vi "check upper bound.vi"(8 "error in (no error)":errorcluster, 9 "ptr upper bound (inclusive)":u64, 10 "size":u64, 11 "ptr in":u64) -> (0 "error out":errorcluster)   [LabVIEW 2018, in "linuxSharedMemory.lvlib"]
uses:
  linuxSharedMemory.lvlib
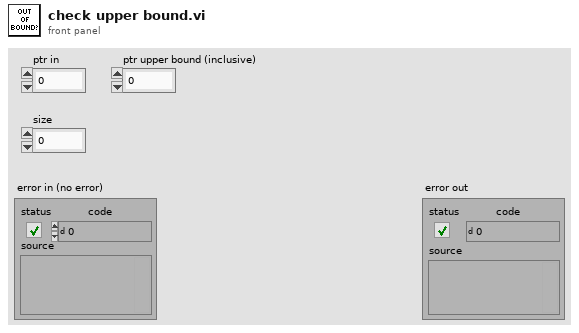
[diagram p1: front panel]
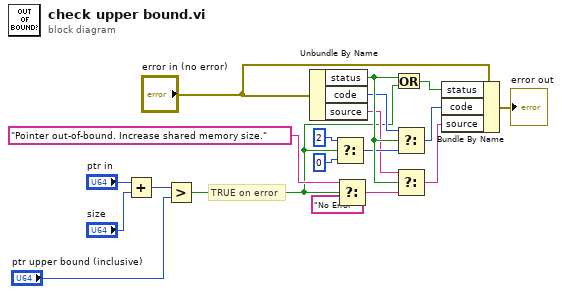
[diagram p0: block diagram]
diagram:
  # "TRUE on error"
  n1 = Add(x="ptr in", y="size") -> (x+y=w3:u64)
  n2 = Greater?(x=w3, y="ptr upper bound (inclusive)") -> (0:w1:bool)
  n3 = Unbundle By Name("error in (no error)") -> ("status"=w11:bool, "code"=w6:i32, "source"=w4:string)
  n4 = Select(t=2, s=w1, f=0) -> (s? t:f=w7:i32)
  n5 = Select(t="Pointer out-of-bound. Increase shared memory size.", s=w1, f="No Error") -> (s? t:f=w5:string)
  n6 = Or(x=w11, y=w1) -> (x .or. y?=w10:bool)
  n7 = Select(t=w6, s=w11, f=w7) -> (s? t:f=w13:i32)
  n8 = Select(t=w4, s=w11, f=w5) -> (s? t:f=w12:string)
  n9 = Bundle By Name(cluster="error in (no error)", "status"=w10, "code"=w13, "source"=w12) -> (→"error out":errorcluster)
